vi "Write Time and Date Info.vi"(6 "Error In":errorcluster, 9 "File Refnum In":refnum<file>) -> (0 "Error Out":errorcluster, 3 "File Refnum Out":refnum<file>)   [LabVIEW 2014]
doc: "The VI auto-generates a string based on date and time and opens a file using the date time string as a file name. An array containing a sine and square wave is converted to a tab delimited string and written to the file. The file is then closed."
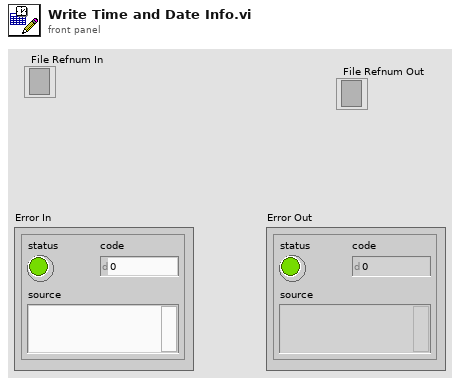
[diagram p1: front panel]
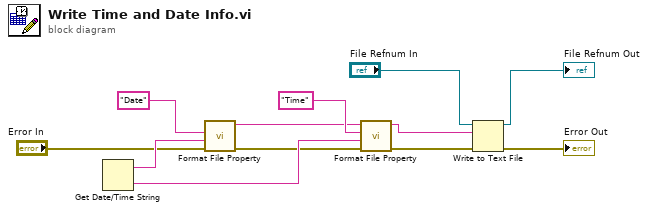
[diagram p0: block diagram]
diagram:
  n1 = Get Date/Time String() -> (date string=w11:string, time string=w8:string)  [unwired: 3 in]
  n2 = call "Format File Property.vi"("Error In"="Error In", "File Property Value"=w11, "File Property Name"="Date") -> ("Error Out"=w7:errorcluster, "String out"=w9:string)  [unwired: 7 in]
  n3 = call "Format File Property.vi"("Error In"=w7, "File Property Value"=w8, "File Property Name"="Time", "String in"=w9) -> ("Error Out"=w2:errorcluster, "String out"=w1:string)  [unwired: 6 in]
  n4 = Write to Text File(file (use dialog)="File Refnum In", text=w1, error in=w2) -> (refnum out=→"File Refnum Out":refnum<file>, error out=→"Error Out":errorcluster)  [unwired: 1 in, 1 out]
